vi "GenerateOccurrence.vi"() -> (3 "Occurrence":i32)   [LabVIEW 2011]
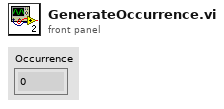
[diagram p1: front panel]
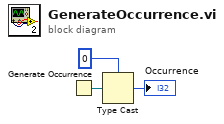
[diagram p0: block diagram]
diagram:
  n1 = Generate Occurrence() -> (w3:refnum<k4>)
  n2 = Type Cast(type=0, x=w3) -> (*(type *) &x=→"Occurrence":i32)
